vi "H5LTdtype_to_text.vi"(6 "error in (no error)":errorcluster, 9 "HDF5 Type Ref":T1) -> (0 "error out":errorcluster, 2 "Text Description":string, 3 "HDF5 Type Ref out":T1)   [LabVIEW 2017]
doc: "Creates a text description of an HDF5 datatype."
uses:
  <vilib>/UPVI/lvhdf5/library.llb/HDF5 Ref.ctl
  <vilib>/UPVI/lvhdf5/hdf5_hl.dll
panel:
  # "LVHDF5 Toolkit\nCopyright (c) 2005-2013 by Jason D. Sommerville\nCopyright (c) 2014 by UPVI, LLC.\n\nThis use and distribution of this file is governed by the terms found in \nLICENSE.txt distributed with this toolkit and installed at\n <user.lib>\\_lvhdf5\\LICENSE.txt"
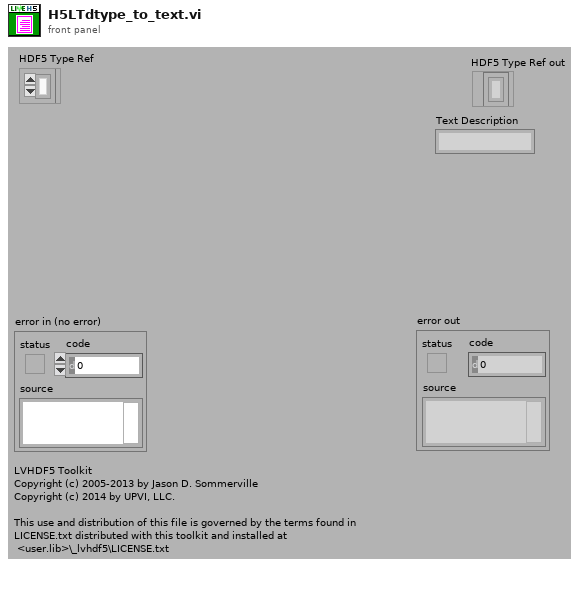
[diagram p1: front panel]
types:
  T1 = typedef "HDF5 Ref.ctl" = refnum<k1>
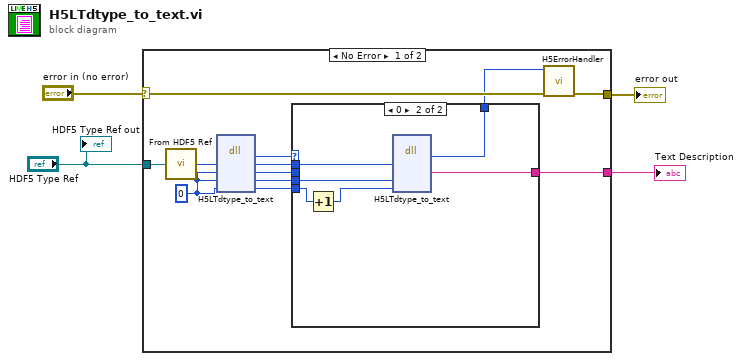
[diagram p0: block diagram]
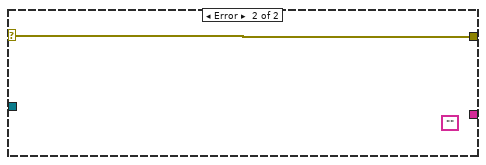
[diagram p3: hidden frame]
diagram:
  n1 = case shown="No Error" "error in (no error)" {
    selector: "error in (no error)" -> [w16 w24]
    tunnel: [w15 w24] -> w3
    tunnel: "HDF5 Type Ref" -> [w14 _]
    tunnel: [w6 _] -> w1
    frame No Error {
      w5 = u32 0
      n2 = call <vilib>:"From HDF5 Ref.vi"("HDF5 Ref"=w14) -> ("I32"=w13:i32)
      n3 = dll-call lib="C:/Program Files/National Instruments/LabVIEW 2017/vi.lib/UPVI/lvhdf5/hdf5_hl.dll" fn="H5LTdtype_to_text"("type_id"=w13, "str"=w5, "lang"=w5, "len"=w5) -> ("return type"=w12:i32, "type_id"=w10:i32, "str"=w9:u64, "lang"=w8:u32, "len"=w7:u32)  [unwired: 3 in, 2 out]
      n4 = case shown="0" w12 {
        selector: w12 -> [w17 _]
        tunnel: [w17 w23] -> w11
        tunnel: w10 -> [_ w22]
        tunnel: w9 -> [_ _]
        tunnel: w8 -> [_ w21]
        tunnel: w7 -> [_ w20]
        tunnel: [_ w18] -> w6
        frame -1, Default {
        }
        frame 0 {
          n5 = Increment(x=w20) -> (x+1=w19:u32)
          n6 = dll-call lib="C:/Program Files/National Instruments/LabVIEW 2017/vi.lib/UPVI/lvhdf5/hdf5_hl.dll" fn="H5LTdtype_to_text"("type_id"=w22, "lang"=w21, "len"=w19) -> ("return type"=w23:i32, "str"=w18:string)  [unwired: 7 in, 2 out]
        }
      }
      n7 = call <vilib>:"H5ErrorHandler.vi"("error in (no error)"=w16, "herr_t"=w11) -> ("error out"=w15:errorcluster)  [unwired: 3 in, 4 out]
    }
    frame Error {
      (unwired) ""
    }
  }
  "error out" <- w3
  "Text Description" <- w1
  "HDF5 Type Ref out" <- "HDF5 Type Ref"
